vi "Get_T-from-interpol.vi"() -> ()   [LabVIEW 2010]
uses:
  CryoTUM_Mischer_Version_2-0/Instrument_Setup.vi
  <vilib>/gmath/NI_Gmath.lvlib
panel:
  out "T(R) interpoliert":dbl[](array[numeric])
  in  "Resistance (Ohm)":dbl
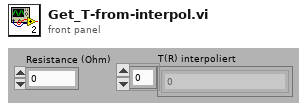
[diagram p1: front panel]
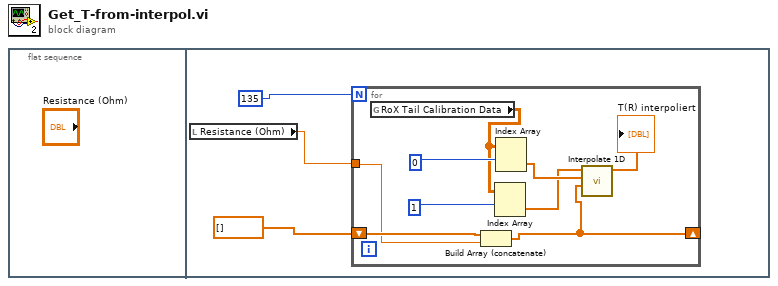
[diagram p0: block diagram]
diagram:
  n1 = flat-sequence {
    frame #0 {
    }
    frame #1 {
      n2 = local read "Resistance (Ohm)"() -> (w1:dbl)
      n3 = for {
        N: 135 -> [_]
        shift-right: [w8] -> _
        shift-left: dbl[] [] -> [w9]
        tunnel: w1 -> [w5]
        n4 = global read "Instrument_Setup.vi" "RoX Tail Calibration Data"() -> (w10:dbl[][])
        n5 = Build Array (concatenate)(w9, w5) -> (w8:dbl[])
        n6 = Index Array(array=w10, index (row)=1) -> (element=w6:dbl[])  [unwired: 1 in]
        n7 = Index Array(array=w10, index (row)=0) -> (element=w7:dbl[])  [unwired: 1 in]
        n8 = call <vilib>:"Interpolate 1D.vi"("xi"=w8, "X"=w7, "Y"=w6) -> ("yi"=→"T(R) interpoliert":dbl[])  [unwired: 6 in, 2 out]
      }
    }
  }
